vi "Insert Sub Panels.vi"(8 "error in (no error)":errorcluster, 9 "Shutdown Event":refnum<user-event>, 10 "Sub Panels":T1, 11 "Owning VI":refnum<vi>) -> (0 "error out":errorcluster)   [LabVIEW 2020, in "User Interface.lvlib"]
doc: "Starts and inserts each sub panel VI into its corresponding sub panel."
uses:
  User Interface.lvlib
  Sub Panels Cluster.ctl
  Sub Panels/Mixing Interface.vi
  Sub Panels/Audio Config.vi
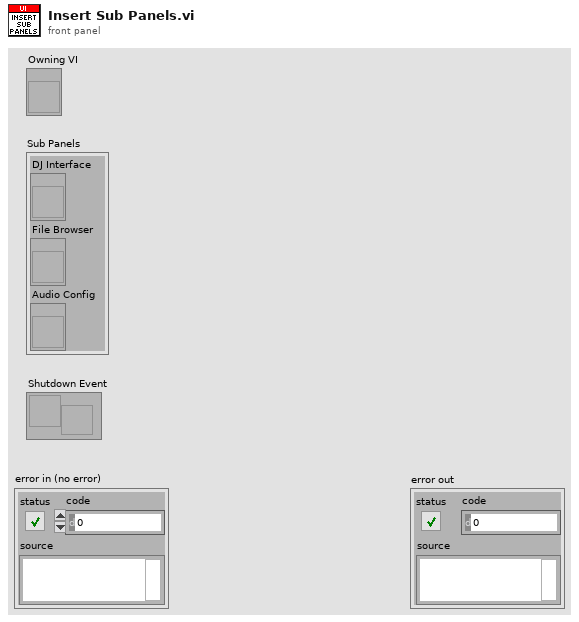
[diagram p1: front panel]
types:
  T1 = typedef "User Interface.lvlib/Sub Panels Cluster.ctl" = cluster{"DJ Interface":refnum<vi>, "File Browser":refnum<vi>, "Audio Config":refnum<vi>}
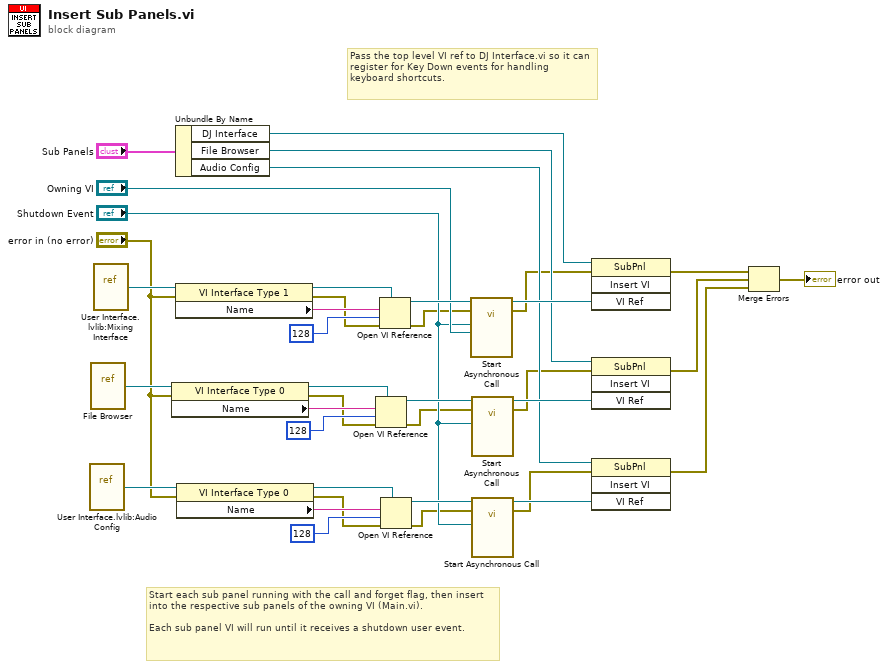
[diagram p0: block diagram]
diagram:
  # "Pass the top level VI ref to DJ Interface.vi so it can register for Key Down events for handling keyboard shortcuts."
  # "Start each sub panel running with the call and forget flag, then insert into the respective sub panels of the owning VI (Main.vi).\n\nEach sub panel VI will run until it receives a shutdown user event."
  n1 = vi-ref "User Interface.lvlib:Audio Config.vi"() -> (w29:refnum<vi>)
  n2 = vi-ref "File Browser.vi"() -> (w38:refnum<vi>)
  n3 = vi-ref "User Interface.lvlib:Mixing Interface.vi"() -> (w28:refnum<vi>)
  n4 = property class="VI Interface Type 0"(reference=w38, error in="error in (no error)") -> (reference out=w36:refnum<vi>, error out=w7:errorcluster, "Name"=w37:string)
  n5 = Unbundle By Name("Sub Panels") -> ("DJ Interface"=w21:refnum<vi>, "File Browser"=w19:refnum<vi>, "Audio Config"=w17:refnum<vi>)
  n6 = property class="VI Interface Type 1"(reference=w28, error in="error in (no error)") -> (reference out=w26:refnum<vi>, error out=w8:errorcluster, "Name"=w27:string)
  n7 = property class="VI Interface Type 0"(reference=w29, error in="error in (no error)") -> (reference out=w31:refnum<vi>, error out=w6:errorcluster, "Name"=w30:string)
  n8 = Open VI Reference(type specifier VI Refnum (for type only)=w36, vi path=w37, options=128, error in (no error)=w7) -> (vi reference=w35:refnum<vi>, error out=w12:errorcluster)  [unwired: 2 in]
  n9 = Open VI Reference(type specifier VI Refnum (for type only)=w26, vi path=w27, options=128, error in (no error)=w8) -> (vi reference=w25:refnum<vi>, error out=w14:errorcluster)  [unwired: 2 in]
  n10 = Open VI Reference(type specifier VI Refnum (for type only)=w31, vi path=w30, options=128, error in (no error)=w6) -> (vi reference=w32:refnum<vi>, error out=w10:errorcluster)  [unwired: 2 in]
  n11 = call-by-ref "Start Asynchronous Call"(reference=w25, error in=w14, "Owning VI"="Owning VI", "Shutdown Event"="Shutdown Event") -> (reference out=w20:refnum<vi>, error out=w13:errorcluster)  [unwired: 10 in]
  n12 = call-by-ref "Start Asynchronous Call"(reference=w35, error in=w12, "Shutdown Event"="Shutdown Event") -> (reference out=w18:refnum<vi>, error out=w11:errorcluster)  [unwired: 11 in]
  n13 = call-by-ref "Start Asynchronous Call"(reference=w32, error in=w10, "Shutdown Event"="Shutdown Event") -> (reference out=w15:refnum<vi>, error out=w9:errorcluster)  [unwired: 11 in]
  n14 = invoke class="SubPnl" method="Insert VI"(reference=w21, error in=w13, "VI Ref"=w20) -> (error out=w5:errorcluster)  [unwired: 1 in, 3 out]
  n15 = invoke class="SubPnl" method="Insert VI"(reference=w19, error in=w11, "VI Ref"=w18) -> (error out=w4:errorcluster)  [unwired: 1 in, 3 out]
  n16 = invoke class="SubPnl" method="Insert VI"(reference=w17, error in=w9, "VI Ref"=w15) -> (error out=w3:errorcluster)  [unwired: 1 in, 3 out]
  n17 = Merge Errors(w5, w4, w3) -> (→"error out":errorcluster)
